vi "Warning.vi"() -> ()   [LabVIEW 2017, in "Assertions.Tests.lvlib" / "Assert Not Error.lvlib"]
uses:
  Assert Not Error.lvlib
  <vilib>/Utility/error.llb/Error Cluster From Error Code.vi
  <vilib>/ErrorRing/Error Ring.xnode
  src/Transparent Assertions/Assertions/Assertions.lvlib
panel:
  out "error out":errorcluster
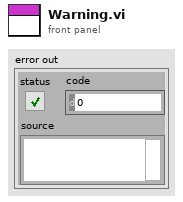
[diagram p1: front panel]
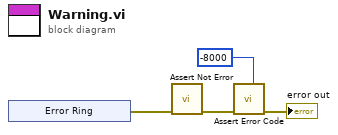
[diagram p0: block diagram]
diagram:
  n1 = xnode "Error Ring"() -> ("error out"=w4:errorcluster)
  n2 = call "Assert Not Error.vi"("error in (no error)"=w4) -> ("error out"=w1:errorcluster)  [unwired: 10 in]
  n3 = call "Assert Error Code.vi"("Expected"=-8000, "error in (no error)"=w1) -> ("error out"=→"error out":errorcluster)  [unwired: 9 in]
